vi "Get NI_XNET_CAN_Bus_Monitor_API SetStreamingFilter Request.vi"(8 "error in (no error)":errorcluster, 11 "gRPCid":T1) -> (0 "error out":errorcluster, 2 "Message Data":T2, 3 "gRPCid out":T1)   [LabVIEW 2025, in "xnet_can_bus_monitor_api_server.lvlib" / "NI_XNET_CAN_Bus_Monitor_API.lvclass"]
uses:
  NI_XNET_CAN_Bus_Monitor_API.lvclass
  RPC Messages/ni_xnet_can_bm_api_SetStreamingFilterRequest.ctl
  RPC Messages/ni_xnet_can_bm_api_FilterInfo.ctl
  RPC Messages/ni_xnet_can_bm_api_DirectionFilter.ctl
  RPC Messages/ni_xnet_can_bm_api_FrameFilter.ctl
  <vilib>/gRPC/LabVIEW gRPC Library/Shared/grpcId.ctl
  NI_XNET_CAN_Bus_Monitor_API.lvclass/NI_XNET_CAN_Bus_Monitor_API.ctl
  xnet_can_bus_monitor_api_server.lvlib
  <vilib>/gRPC/LabVIEW gRPC Library/grpc-lvsupport-release.lvlib
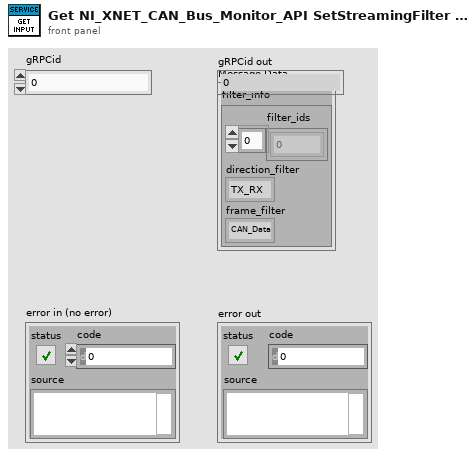
[diagram p1: front panel]
types:
  T1 = typedef "grpc-lvsupport-release.lvlib/grpcId.ctl" = u64
  T2 = typedef "xnet_can_bus_monitor_api_server.lvlib/ni_xnet_can_bm_api_SetStreamingFilterRequest.ctl" = cluster{"filter_info":T3}
  T3 = typedef "xnet_can_bus_monitor_api_server.lvlib/ni_xnet_can_bm_api_FilterInfo.ctl" = cluster{"filter_ids":u32[], "direction_filter":T4, "frame_filter":T5}
  T4 = typedef "xnet_can_bus_monitor_api_server.lvlib/ni_xnet_can_bm_api_DirectionFilter.ctl" = enum32{"TX_RX", "RX", "TX"}
  T5 = typedef "xnet_can_bus_monitor_api_server.lvlib/ni_xnet_can_bm_api_FrameFilter.ctl" = enum32{"CAN_Data", "CAN_Remote", "CAN_Bus_Error", "CAN_2_Data", "CAN_FD_Data", "CAN_FD_BRS_Data", "J1939_Data", "Delay", "Log_Trigger", "Start_Trigger", "All"}
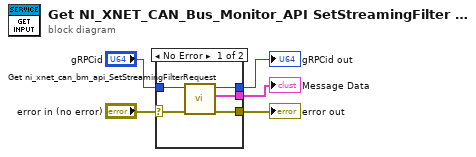
[diagram p0: block diagram]
diagram:
  n1 = case shown="No Error" "error in (no error)" {
    selector: "error in (no error)" -> [w10 w12]
    tunnel: [w9 w12] -> w4
    tunnel: [w8 _] -> w3
    tunnel: "gRPCid" -> [w7 w11]
    tunnel: [w6 w11] -> w1
    frame No Error {
      n2 = call "Get ni_xnet_can_bm_api_SetStreamingFilterRequest.vi"("error in (no error)"=w10, "gRPCid"=w7) -> ("error out"=w9:errorcluster, "package_templatemessage"=w8:T2, "gRPCid out"=w6:T1)  [unwired: 7 in]
    }
    frame Error {
    }
  }
  "error out" <- w4
  "Message Data" <- w3
  "gRPCid out" <- w1
